vi "Launch Broker.vi"(8 "error in":errorcluster, 11 "System in":refnum<class "System.lvclass">) -> (0 "error out":errorcluster, 3 "System out":refnum<class "System.lvclass">)   [LabVIEW 2014, in "System.lvclass"]
uses:
  System.lvclass
  Broker_class/Broker.lvclass
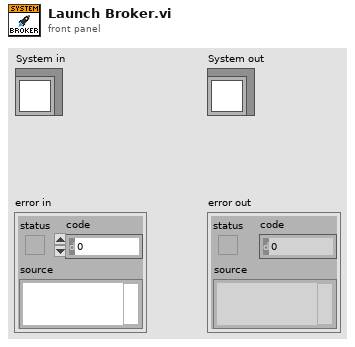
[diagram p1: front panel]
types:
  T1 = typedef "Topic Ref.ctl" = cluster{"Name":string, "Path":path, "Subscribers":string[]}
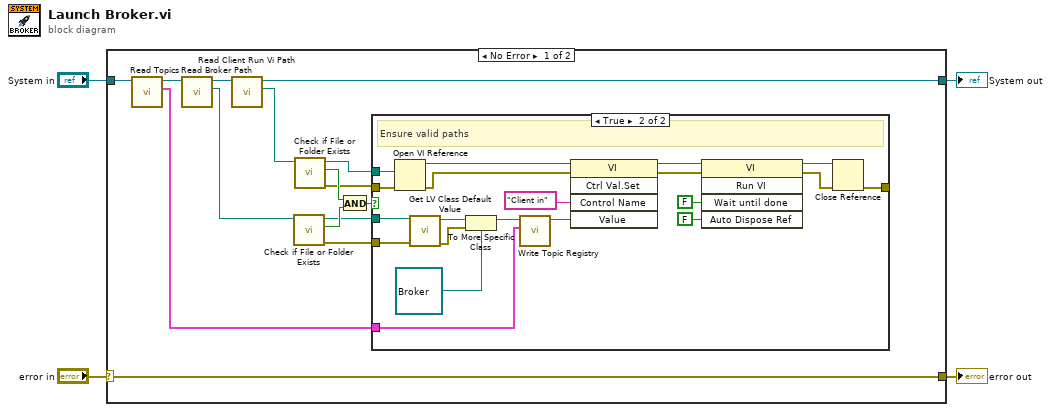
[diagram p0: block diagram]
diagram:
  n1 = case shown="No Error" "error in" {
    selector: "error in" -> [w19 w42]
    tunnel: [w19 w42] -> w1
    tunnel: [w11 w41] -> w3
    tunnel: "System in" -> [w9 w41]
    frame No Error {
      n2 = call-dynamic "Read Topics.vi"("System in"=w9) -> ("Topics"=w8:T1[], "System out"=w7:refnum<class "System.lvclass">)  [unwired: 8 in, 1 out]
      n3 = call-dynamic "Read Broker Path.vi"("System in"=w7) -> ("Broker Path"=w5:path, "System out"=w6:refnum<class "System.lvclass">)  [unwired: 8 in, 1 out]
      n4 = call-dynamic "Read Client Run Vi Path.vi"("System in"=w6) -> ("Client Run Vi Path"=w10:path, "System out"=w11:refnum<class "System.lvclass">)  [unwired: 8 in, 1 out]
      n5 = call <vilib>:"Check if File or Folder Exists.vi"("path"=w5) -> ("error out"=w13:errorcluster, "file or folder exists?"=w17:bool, "dup path"=w12:path)  [unwired: 8 in]
      n6 = call <vilib>:"Check if File or Folder Exists.vi"("path"=w10) -> ("error out"=w15:errorcluster, "file or folder exists?"=w16:bool, "dup path"=w14:path)  [unwired: 8 in]
      n7 = And(x=w16, y=w17) -> (x .and. y?=w18:bool)
      n8 = case shown="True" w18 {
        tunnel: w12 -> [_ w36]
        tunnel: w13 -> [w20 w35]
        tunnel: [w20 w38] -> _
        tunnel: w14 -> [_ w33]
        tunnel: w15 -> [_ w32]
        tunnel: w8 -> [_ w21]
        frame False {
        }
        frame True {
          # "Ensure valid paths"
          n9 = Open VI Reference(vi path=w33, error in (no error)=w32) -> (vi reference=w26:refnum<vi>, error out=w25:errorcluster)  [unwired: 4 in]
          n10 = call <vilib>:"Get LV Class Default Value.vi"("error in (no error)"=w35, "class path"=w36) -> ("error out"=w34:errorcluster, "object"=w37:refnum<class>)  [unwired: 8 in]
          n11 = To More Specific Class(target class=refnum<class "Broker.lvclass"> refnum ("Broker.lvclass"), reference=w37, error in=w34) -> (specific class reference=w23:refnum<class "Broker.lvclass">)  [unwired: 1 out]
          n12 = call-dynamic "Write Topic Registry.vi"("Topic Registry"=w21, "Broker in"=w23) -> ("Broker out"=w22:refnum<class "Broker.lvclass">)  [unwired: 8 in, 1 out]
          n13 = invoke class="VI" method="Ctrl Val.Set"(reference=w26, error in=w25, "Control Name"="Client in" ("Client Name"), "Value"=w22) -> (reference out=w29:refnum<vi>, error out=w28:errorcluster)  [unwired: 1 in, 3 out]
          n14 = invoke class="VI" method="Run VI"(reference=w29, error in=w28, "Wait until done"=FALSE ("Wait Until Done"), "Auto Dispose Ref"=FALSE ("Auto Dispose Reference")) -> (reference out=w40:refnum<vi>, error out=w39:errorcluster)  [unwired: 1 in, 3 out]
          n15 = Close Reference(reference=w40, error in (no error)=w39) -> (error out=w38:errorcluster)
        }
      }
    }
    frame Error {
    }
  }
  "error out" <- w1
  "System out" <- w3
